vi "RSNRPZ Set Scope Measurements Level Thresholds.vi"(6 "Transition Low Ref (10.0 %)":dbl=10.0 format="%^.3e", 7 "Transition High Ref (90.0 %)":dbl=90.0 format="%^.3e", 8 "error in (no error)":errorcluster, 9 "Duration Ref (50.0 %)":dbl=50.0 format="%^.3e", 10 "Channel (1)":i32=1, 11 "VISA session":refnum<visa-resource-name> caption="VISA resource name") -> (0 "error out":errorcluster, 3 "dup VISA session":refnum<visa-resource-name> caption="VISA resource name")   [LabVIEW 2010]
doc: "This VI defines the thresholds of the reference and transition levels that are used for the calculation of the pulse's time parameter.\nThe duration reference level is used to calculate pulse duration and pulse period, the transition low and high levels are used to calculate the pulse transition’s rise/fall time and their occurrences.\n\nNote:\n1) This VI is only available for NRP-Z81.\n\nRemote-control command(s):\nSENS:TRAC:MEAS:DEF:DUR:REF \nSENS:TRAC:MEAS:DEF:TRAN:LREF\nSENS:TRAC:MEAS:DEF:TRAN:HREF"
uses:
  rsnrpz_32.dll
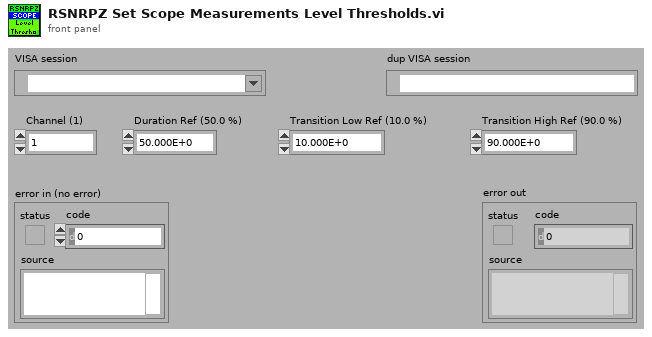
[diagram p1: front panel]
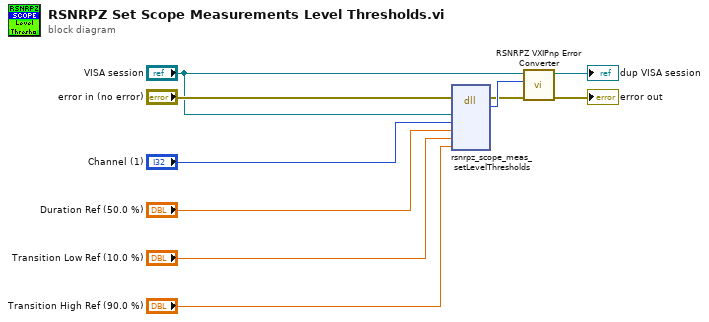
[diagram p0: block diagram]
diagram:
  n1 = dll-call lib="rsnrpz_32.dll" fn="rsnrpz_scope_meas_setLevelThresholds"(error in="error in (no error)", "Instrument Handle"="VISA session", "Channel"="Channel (1)", "Duration Ref"="Duration Ref (50.0 %)", "Transition Low Ref"="Transition Low Ref (10.0 %)", "Transition High Ref"="Transition High Ref (90.0 %)") -> (error out=w5:errorcluster, "Status"=w10:i32)  [unwired: 7 in, 1 out]
  n2 = call <instrlib>:"RSNRPZ VXIPnp Error Converter.vi"("error in"=w5, "VXIPnp error code"=w10, "VISA session"="VISA session") -> ("error out"=→"error out":errorcluster, "dup VISA session"=→"dup VISA session":refnum<visa-resource-name>)  [unwired: 7 in]
